vi "test_Bitfile Reload_Bitpacked Group Scalars Data Type Change.vi"(8 "error in (no error)":errorcluster, 11 "TestCase in":refnum<class "FPGA Addon Bitfile Reload Unit Tests.lvclass">=refnum) -> (0 "error out":errorcluster, 3 "TestCase out":refnum<class "FPGA Addon Bitfile Reload Unit Tests.lvclass">)   [LabVIEW 2026, in "FPGA Addon Bitfile Reload Unit Tests.lvclass"]
uses:
  FPGA Addon Bitfile Reload Unit Tests.lvclass
  APIs/Scripting API/TypeDefs/Output Scalar Data.ctl
  APIs/Scripting API/Scripting API.lvlib
  FPGA Addon Test Class/FPGA Addon Test Class.lvclass
  Addon/Addon System Explorer/FPGA Addon System Explorer.lvlib
  Addon/Addon Shared/SubVIs/Constants.vi
  Addon/Addon Shared/FPGA Addon Shared.lvlib
  Addon/Addon Shared/Types/FPGA Addon Data Type.ctl
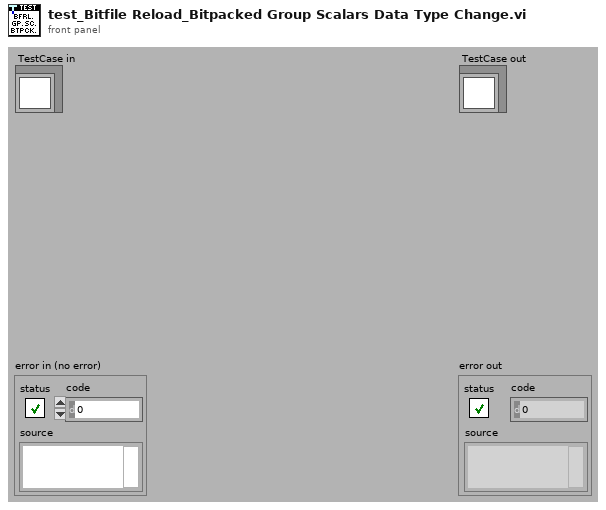
[diagram p1: front panel]
types:
  T1 = typedef "Scripting API.lvlib/Output Scalar Data.ctl" = cluster{"Bitfile Name":string, "SysDef Channel Name":string, "Imported":bool, "Data Type":T2}
  T2 = typedef "FPGA Addon Shared.lvlib/FPGA Addon Data Type.ctl" = enum8{"<Null>", "I8", "I16", "I32", "I64", "U8", "U16", "U32", "U64", "SGL", "Boolean", "Analog PWM In Settings", "Analog PWM In", "Digital PWM In Settings", "Digital PWM In", "Digital PWM Out", "Sine Out", "FXP", "FXP+/-24.5", "FXP+/-16.5", "FXP+/-32.8", "FXP+/-64.32", "FXP+/-16.7", "FXP+/-20.5", "FXP+/-27.5", "FXP+/-32.16", "FXP+16.3", "FXP+18.3", "Digital Static In", "Digital Static Out", "Digital Static In Settings", "Digital WSS Out", "Quad Encoder Settings", "Quad Encoder In", "Group"}
  T3 = typedef "Custom Device API.lvlib/Custom Device Item Ref.ctl" = u64
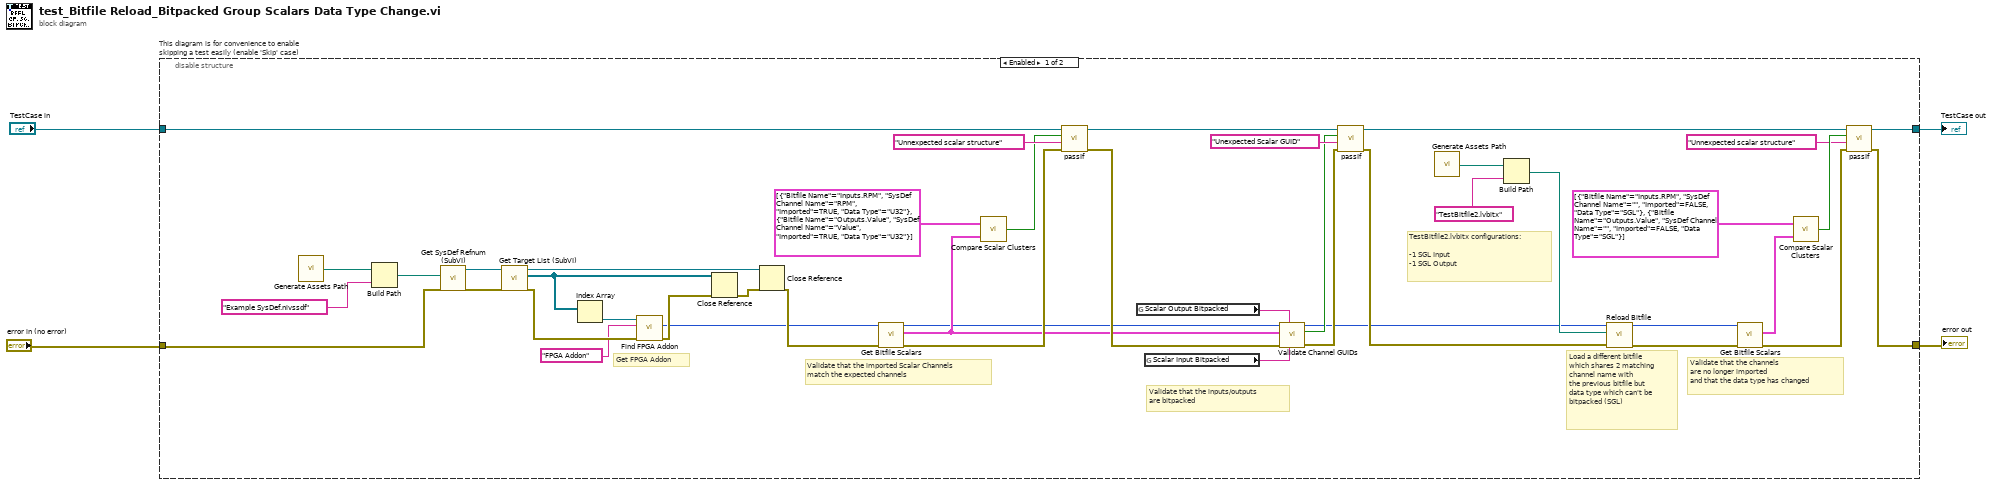
[diagram p0: block diagram]
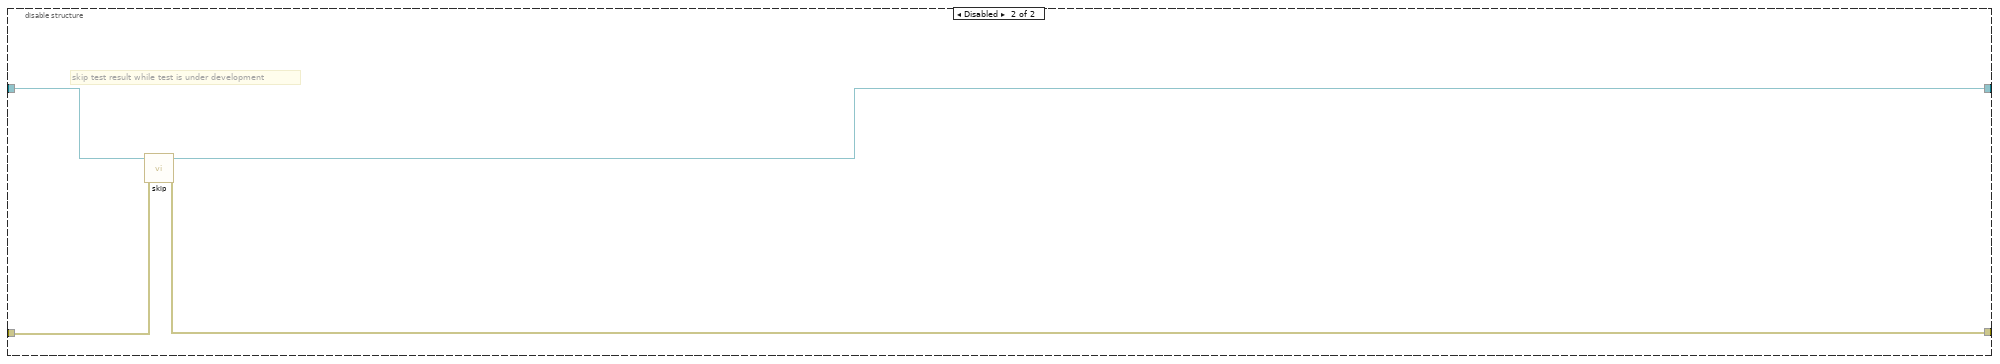
[diagram p2: hidden frame]
diagram:
  n1 = disable-structure "This diagram is for convenience to enable skipping a test easily (enable 'Skip' case)" shown="Enabled" {
    disable-tunnel: "TestCase in" -> [w29 w52]
    disable-tunnel: [w27 w50] -> w1
    disable-tunnel: [w26 w51] -> w3
    disable-tunnel: "error in (no error)" -> [w28 w49]
    frame Enabled {
      # "Validate that the inputs/outputs \nare bitpacked"
      # "TestBitfile2.lvbitx configurations:\n\n-1 SGL Input\n-1 SGL Output"
      # "Validate that the channels \nare no longer imported \nand that the data type has changed"
      # "Load a different bitfile\nwhich shares 2 matching\nchannel name with \nthe previous bitfile but \ndata type which can't be\nbitpacked (SGL)"
      # "Validate that the imported Scalar Channels\nmatch the expected channels"
      # "Get FPGA Addon"
      n2 = call "Generate Assets Path.vi"() -> ("Assets path"=w40:path)
      n3 = Build Path(base path=w40, name or relative path="Example SysDef.nivssdf") -> (appended path=w47:path)
      n4 = call "Get SysDef Refnum (SubVI).vi"("error in (no error)"=w28, "System Definition path"=w47) -> ("error out"=w45:errorcluster, "NationalInstruments.VeriStand.SystemDefinitionAPI.SystemDefinition"=w46:refnum<k39>)  [unwired: 8 in]
      n5 = call "Get Target List (SubVI).vi"("error in (no error)"=w45, "NationalInstruments.VeriStand.SystemDefinitionAPI.SystemDefinition"=w46) -> ("error out"=w25:errorcluster, "Target List Refnums"=w44:refnum<k39>[], "NationalInstruments.VeriStand.SystemDefinitionAPI.SystemDefinition"=w43:refnum<k39>)  [unwired: 7 in]
      n6 = Index Array(array=w44) -> (element=w24:refnum<k39>)  [unwired: 1 in]
      n7 = call "Find FPGA Addon.vi"("error in"=w25, "FPGA addon name"="FPGA Addon", "NationalInstruments.VeriStand.SystemDefinitionAPI.Target"=w24) -> ("error out"=w22:errorcluster, "FPGA addon refnum out"=w20:T3)  [unwired: 5 in, 2 out]
      n8 = Close Reference(reference=w44, error in (no error)=w22) -> (error out=w42:errorcluster)
      n9 = Close Reference(reference=w43, error in (no error)=w42) -> (error out=w21:errorcluster)
      n10 = call "Get Bitfile Scalars.vi"("error in"=w21, "FPGA addon refnum in"=w20) -> ("error out"=w19:errorcluster, "bitfile scalars out"=w11:T1[], "FPGA addon refnum out"=w10:T3)  [unwired: 7 in]
      n11 = call "Compare Scalar Clusters.vi"("Target bitfile scalars in"=w11, "Reference bitfile scalars in"=T1[] [{"Bitfile Name"="Inputs.RPM", "SysDef Channel Name"="RPM", "Imported"=TRUE, "Data Type"=enum."U32"}, {"Bitfile Name"="Outputs.Value", "SysDef Channel Name"="Value", "Imported"=TRUE, "Data Type"=enum."U32"}] ("bitfile scalars out")) -> ("Equal ?"=w39:bool)
      n12 = call-dynamic "passIf.vi"("error in (no error)"=w19, "message (\"\")"="Unnexpected scalar structure" ("message (\"\")"), "pass"=w39, "TestCase in"=w29) -> ("error out"=w12:errorcluster, "TestCase out"=w18:refnum<class "FPGA Addon Bitfile Reload Unit Tests.lvclass">)  [unwired: 6 in]
      n13 = global read "Constants.vi" "Scalar Output Bitpacked"() -> (w5:string)
      n14 = global read "Constants.vi" "Scalar Input Bitpacked"() -> (w6:string)
      n15 = call "Validate Channel GUIDs.vi"("input GUID"=w6, "output GUID"=w5, "error in (no error)"=w12, "imported bitfile scalars in"=w11, "FPGA addon refnum in"=w10) -> ("error out"=w9:errorcluster, "valid GUIDs?"=w8:bool, "FPGA addon refnum out"=w7:T3)  [unwired: 4 in]
      n16 = call-dynamic "passIf.vi"("error in (no error)"=w9, "message (\"\")"="Unexpected Scalar GUID" ("message (\"\")"), "pass"=w8, "TestCase in"=w18) -> ("error out"=w16:errorcluster, "TestCase out"=w15:refnum<class "FPGA Addon Bitfile Reload Unit Tests.lvclass">)  [unwired: 6 in]
      n17 = call "Generate Assets Path.vi"() -> ("Assets path"=w37:path)
      n18 = Build Path(base path=w37, name or relative path="TestBitfile2.lvbitx") -> (appended path=w36:path)
      n19 = call "Reload Bitfile.vi"("error in (no error)"=w16, "NewVal"=w36, "Item Ref in"=w7) -> ("error out"=w35:errorcluster, "Section Ref out"=w34:T3)  [unwired: 7 in]
      n20 = call "Get Bitfile Scalars.vi"("error in"=w35, "FPGA addon refnum in"=w34) -> ("error out"=w32:errorcluster, "bitfile scalars out"=w33:T1[])  [unwired: 7 in, 1 out]
      n21 = call "Compare Scalar Clusters.vi"("Target bitfile scalars in"=w33, "Reference bitfile scalars in"=T1[] [{"Bitfile Name"="Inputs.RPM", "SysDef Channel Name"="", "Imported"=FALSE, "Data Type"=enum."SGL"}, {"Bitfile Name"="Outputs.Value", "SysDef Channel Name"="", "Imported"=FALSE, "Data Type"=enum."SGL"}] ("bitfile scalars out 2")) -> ("Equal ?"=w31:bool)
      n22 = call-dynamic "passIf.vi"("error in (no error)"=w32, "message (\"\")"="Unnexpected scalar structure" ("message (\"\")"), "pass"=w31, "TestCase in"=w15) -> ("error out"=w26:errorcluster, "TestCase out"=w27:refnum<class "FPGA Addon Bitfile Reload Unit Tests.lvclass">)  [unwired: 6 in]
    }
    frame Disabled {
      # "skip test result while test is under development"
      n23 = call <vilib>:"skip.vi"("error in (no error)"=w49, "TestCase in"=w52) -> ("error out"=w51:errorcluster, "TestCase out"=w50:refnum<class "FPGA Addon Bitfile Reload Unit Tests.lvclass">)  [unwired: 8 in]
    }
  }
  "error out" <- w3
  "TestCase out" <- w1
